vi "设置单元格值.vi"(0 "Excel._Worksheet 2":refnum<k7> caption="Excel._Worksheet", 1 "Row":i32 caption="行", 2 "Col":i32 caption="列", 3 "Value":string caption="值", 4 "error in (no error)":errorcluster caption="错误输入（无错误）") -> (5 "Excel._Worksheet":refnum<k7>, 6 "error out":errorcluster caption="错误输出")   [LabVIEW 2018]
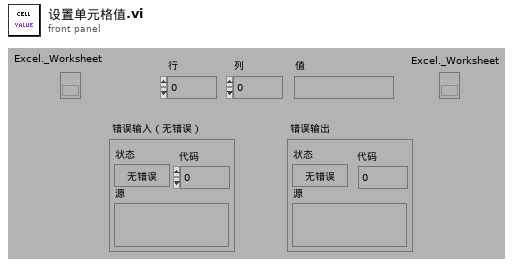
[diagram p1: front panel]
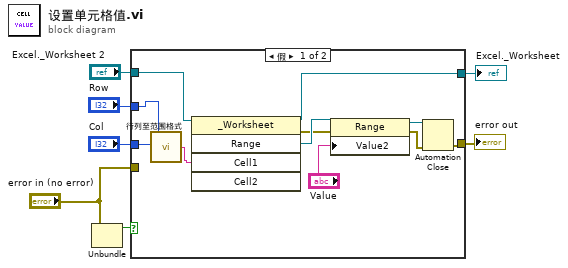
[diagram p0: block diagram]
diagram:
  n1 = Unbundle("error in (no error)") -> ("status"=w5:bool)  [unwired: 2 out]
  n2 = case shown="假" w5 {
    tunnel: "Col" -> [w9 _]
    tunnel: "Row" -> [w10 _]
    tunnel: "error in (no error)" -> [_ w20]
    tunnel: [w13 w20] -> w3
    tunnel: [w12 w19] -> w6
    tunnel: "Excel._Worksheet 2" -> [w11 w19]
    frame False {
      n3 = call "行列至范围格式.vi"("Column"=w9, "row"=w10) -> ("Output String"=w8:string)
      n4 = invoke class="_Worksheet" method="Range"(reference=w11, "Cell1"=w8) -> (reference out=w12:refnum<k7>, error out=w17:errorcluster, "Range"=w18:refnum<k7>)  [unwired: 3 in, 2 out]
      n5 = property class="Range"(reference=w18, error in=w17, "Value2"="Value") -> (reference out=w15:refnum<k7>, error out=w14:errorcluster)
      n6 = Automation Close(3:w14, 5:w15) -> (0:w13:errorcluster)
    }
    frame True {
    }
  }
  "Excel._Worksheet" <- w6
  "error out" <- w3
